vi "GUI Open Synchronization Objects.vi"(8 "error in (no error)":errorcluster) -> (0 "error out":errorcluster, 3 "FOFB GUI":T1)   [LabVIEW 2011, in "User Interface VIs.lvlib"]
uses:
  User Interface VIs.lvlib
  Types Definitions/Type FOFB GUI.ctl
  Types Definitions/Type FOFB Parameters.ctl
  Types Definitions/Type Network Configuration.ctl
  Types Definitions/Type FA Configuration.ctl
  Types Definitions/Type Response Matrix Measurement Configuration.ctl
  Types Definitions/Type Correction Algorithm Configuration.ctl
  Types Definitions/Type Acquisition Network Configuration.ctl
  Types Definitions/Type Actuation Network Configuration.ctl
  Types Definitions/Type Configuration Loop Mode.ctl
  Types Definitions/Type Configuration Data (GUI to Controller).ctl
  Types Definitions/Type Monitoring Data.ctl
  Types Definitions/Type Diagnostics Data.ctl
  Types Definitions/Type CPU Loads Array.ctl
  Types Definitions/Type CPU Loads.ctl
  Types Definitions/Type Diagnostics Sample.ctl
  Types Definitions/Type Monitoring Sample.ctl
  Type Definitions.lvlib
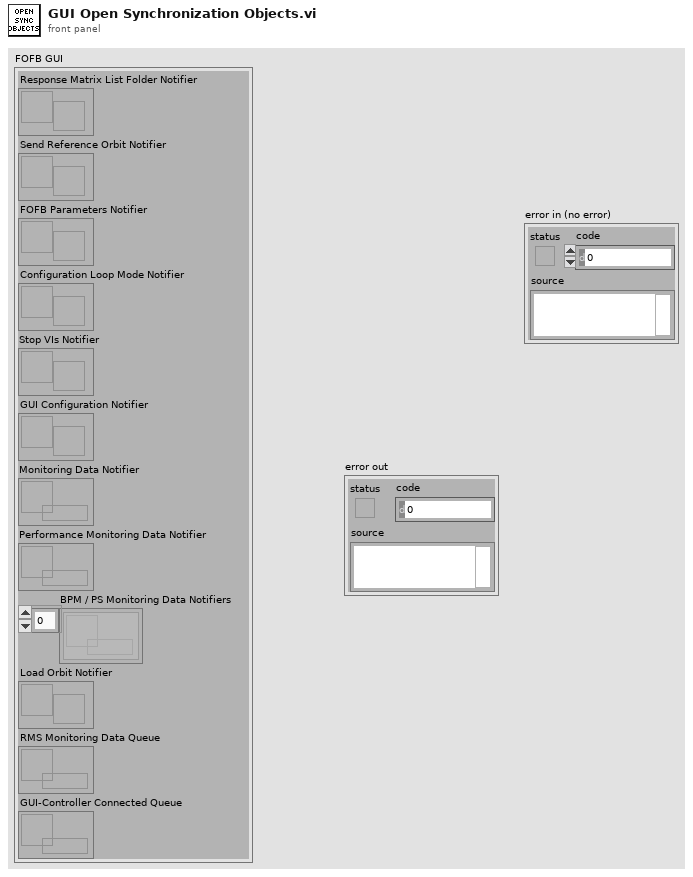
[diagram p1: front panel]
types:
  T1 = typedef "Type Definitions.lvlib/Type FOFB GUI.ctl" = cluster{"Response Matrix List Folder Notifier":refnum<notifier>, "Send Reference Orbit Notifier":refnum<notifier>, "FOFB Parameters Notifier":refnum<notifier>, "Configuration Loop Mode Notifier":refnum<notifier>, "Stop VIs Notifier":refnum<notifier>, "GUI Configuration Notifier":refnum<notifier>, "Monitoring Data Notifier":refnum<queue>, "Performance Monitoring Data Notifier":refnum<queue>, "BPM / PS Monitoring Data Notifiers":refnum<queue>[], "Load Orbit Notifier":refnum<notifier>, "RMS Monitoring Data Queue":refnum<queue>, "GUI-Controller Connected Queue":refnum<queue>}
  T2 = typedef "Type Definitions.lvlib/Type Configuration Loop Mode.ctl" = enum8{"Operation Mode", "Request FOFB Parameters", "Send New FOFB Parameters", "Send Reference Orbit", "Request Response Matrix List Folder"}
  T3 = typedef "Type Definitions.lvlib/Type FOFB Parameters.ctl" = cluster{"Network":T4, "Fast Acquisition":T5, "Response Matrix Measurement":T6, "Correction Algorithm":T7, "Acquisition Network":T8, "Actuation Network":T9}
  T4 = typedef "Type Definitions.lvlib/Type Network Configuration.ctl" = cluster{"FOFB Controller IP":string, "LNLS Control Network IP":string, "LNLS Control Network Power Supplies TCP Port":u16, "LNLS Control Network FOFB Configuration TCP Port":u16, "Data Server TCP Port":u16, "Monitoring Data TCP Port":u16, "Configuration GUI TCP Port":u16, "TCP Listening Timeout":i32}
  T5 = typedef "Type Definitions.lvlib/Type FA Configuration.ctl" = cluster{"Acquisition Period":u32, "Data Buffer Size":u32, "Monitoring Period":u32}
  T6 = typedef "Type Definitions.lvlib/Type Response Matrix Measurement Configuration.ctl" = cluster{"Step Amplitude":dbl, "Time Between Steps":u32, "Step Duration":u32, "Number of Averages":u32}
  T7 = typedef "Type Definitions.lvlib/Type Correction Algorithm Configuration.ctl" = cluster{"Correction Period":u32, "Reference Orbit Path":path, "Response Matrix Path":path, "Correction Matrix Path":path, "Horizontal Correction Factor":dbl, "Vertical Correction Factor":dbl, "Beam Current FOFB Threshold":dbl, "Decouple H-V":bool, "Use Additional BPM LPF":bool, "BPM LPF Cutoff":dbl}
  T8 = typedef "Type Definitions.lvlib/Type Acquisition Network Configuration.ctl" = cluster{"Chassis Name":string, "Variables":cluster{"Variable Name":string, "Matrix Order":u32, "Location":dbl, "Plane":enum8{"H", "V"}, "On Correction":bool}[]}[]
  T9 = typedef "Type Definitions.lvlib/Type Actuation Network Configuration.ctl" = cluster{"Chassis Name":string, "Variables":cluster{"Variable Name":string, "Matrix Order":u32, "RMM Step Factor":dbl, "Plane":enum8{"H", "V"}, "On Correction":bool, "Kc":dbl, "Ti":dbl, "Td":dbl}[]}[]
  T10 = typedef "Type Definitions.lvlib/Type Configuration Data (GUI to Controller).ctl" = cluster{"Update Controller Soft Configuration":bool[], "Request RT Execution Trace":string[], "Reference Orbit":dbl[], "Request Response Matrix Folder List":bool[], "Request FOFB Parameters":bool[], "FOFB Parameters":T3[]}
  T11 = typedef "Type Definitions.lvlib/Type Diagnostics Sample.ctl" = cluster{"Timestamp":timestamp, "Diagnostics Data":T12}
  T12 = typedef "Type Definitions.lvlib/Type Diagnostics Data.ctl" = cluster{"Time-Critical Loop Missed Iterations":u32, "Time-Critical Loop Execution Time (usec)":u32, "FA Buffer Usage":u32, "Available Memory (bytes)":u32, "CPU Loads Array":T13}
  T13 = typedef "Type Definitions.lvlib/Type CPU Loads Array.ctl" = T14[]
  T14 = typedef "Type Definitions.lvlib/Type CPU Loads.ctl" = cluster{"Total (%)":dbl, "Time Critical (%)":dbl, "Timed Structures (%)":dbl, "High (%)":dbl, "Above Normal (%)":dbl, "Normal (%)":dbl, "Background (%)":dbl, "Idle (%)":dbl, "ISR (%)":dbl}
  T15 = typedef "Type Definitions.lvlib/Type Monitoring Sample.ctl" = cluster{"Timestamp":timestamp, "Sample":dbl[]}
  T16 = typedef "Type Definitions.lvlib/Type Monitoring Data.ctl" = cluster{"Timestamp":timestamp, "BPM Readings":dbl[], "PS Readings":dbl[], "PS FOFB Setpoints":dbl[], "PS Status per Rack":u8[], "PS ON-OFF per Rack":u8[], "Operation Mode":enum16{"Idle Mode", "Error Mode", "Manual Mode", "FOFB Mode", "RMM Mode"}, "Diagnostics Data":T12, "Controller Status Table":i32[]}
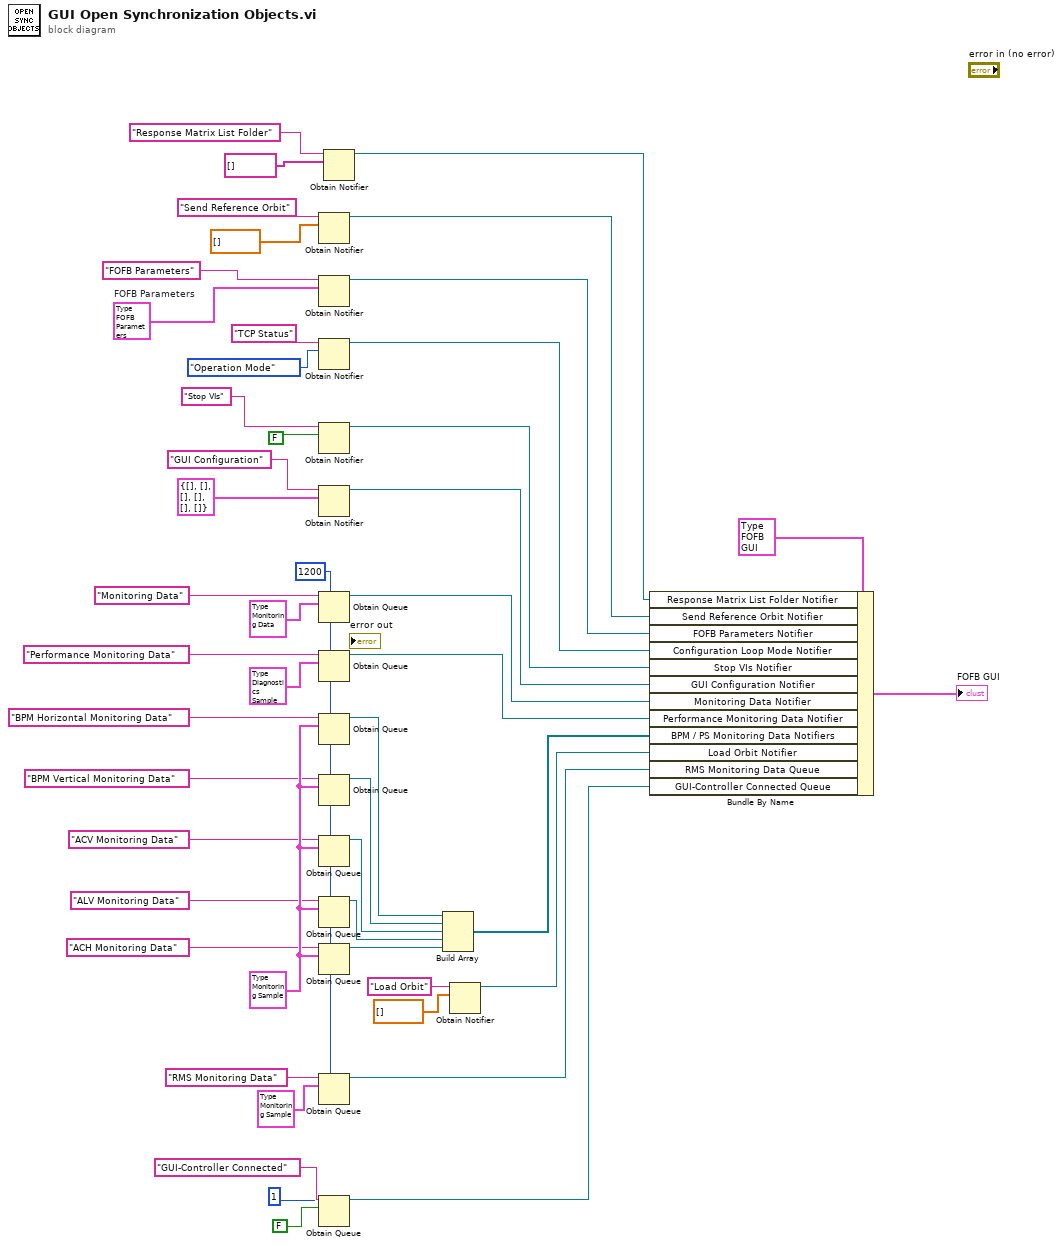
[diagram p0: block diagram]
diagram:
  w10 = T3 {"Network"={"FOFB Controller IP"="", "LNLS Control Network IP"="", "LNLS Control Network Power Supplies TCP Port"=0, "LNLS Control Network FOFB Configuration TCP Port"=0, "Data Server TCP Port"=0, "Monitoring Data TCP Port"=0, "Configuration GUI TCP Port"=0, "TCP Listening Timeout"=0}, "Fast Acquisition"={"Acquisition Period"=0, "Data Buffer Size"=0, "Monitoring Period"=0}, "Response Matrix Measurement"={"Step Amplitude"=0.0, "Time Between Steps"=0, "Step Duration"=0, "Number of Averages"=0}, "Correction Algorithm"={"Correction Period"=0, "Reference Orbit Path"=path "", "Response Matrix Path"=path "", "Correction Matrix Path"=path "", "Horizontal Correction Factor"=0.0, "Vertical Correction Factor"=0.0, "Beam Current FOFB Threshold"=0.0, "Decouple H-V"=FALSE, "Use Additional BPM LPF"=FALSE, "BPM LPF Cutoff"=0.0}, "Acquisition Network"=[], "Actuation Network"=[]}  # FOFB Parameters
  w37 = T15 {"Timestamp"=timestamp(0 s since 1904-01-01), "Sample"=[]} ("Monitoring Sample")
  w13 = 1200 ("max queue size (-1, unlimited)")
  n1 = Obtain Notifier(name (unnamed)="Send Reference Orbit", notification data type=dbl[] [] ("Orbit")) -> (notifier out=w5:refnum<notifier>)  [unwired: 2 in, 2 out]
  n2 = Obtain Notifier(name (unnamed)="FOFB Parameters", notification data type=w10) -> (notifier out=w9:refnum<notifier>)  [unwired: 2 in, 2 out]
  n3 = Obtain Notifier(name (unnamed)="TCP Status", notification data type=Type_Configuration_Loop_Mode."Operation Mode" ("notification")) -> (notifier out=w8:refnum<notifier>)  [unwired: 2 in, 2 out]
  n4 = Obtain Notifier(name (unnamed)="Stop VIs", notification data type=FALSE) -> (notifier out=w41:refnum<notifier>)  [unwired: 2 in, 2 out]
  n5 = Obtain Notifier(name (unnamed)="GUI Configuration", notification data type=T10 {"Update Controller Soft Configuration"=[], "Request RT Execution Trace"=[], "Reference Orbit"=[], "Request Response Matrix Folder List"=[], "Request FOFB Parameters"=[], "FOFB Parameters"=[]} ("Configuration Data (GUI to Controller)")) -> (notifier out=w42:refnum<notifier>)  [unwired: 2 in, 2 out]
  n6 = Obtain Queue(max queue size (-1, unlimited)=w13, name (unnamed)="Monitoring Data", element data type=T16 {"Timestamp"=timestamp(0 s since 1904-01-01), "BPM Readings"=[], "PS Readings"=[], "PS FOFB Setpoints"=[], "PS Status per Rack"=[], "PS ON-OFF per Rack"=[], "Operation Mode"=enum."Idle Mode", "Diagnostics Data"={"Time-Critical Loop Missed Iterations"=0, "Time-Critical Loop Execution Time (usec)"=0, "FA Buffer Usage"=0, "Available Memory (bytes)"=0, "CPU Loads Array"=[]}, "Controller Status Table"=[]} ("Slow Data")) -> (queue out=w43:refnum<queue>)  [unwired: 2 in, 2 out]
  n7 = Obtain Queue(max queue size (-1, unlimited)=w13, name (unnamed)="Performance Monitoring Data", element data type=T11 {"Timestamp"=timestamp(0 s since 1904-01-01), "Diagnostics Data"={"Time-Critical Loop Missed Iterations"=0, "Time-Critical Loop Execution Time (usec)"=0, "FA Buffer Usage"=0, "Available Memory (bytes)"=0, "CPU Loads Array"=[]}} ("Diagnostics  Sample")) -> (queue out=w44:refnum<queue>)  [unwired: 2 in, 2 out]
  n8 = Obtain Queue(max queue size (-1, unlimited)=w13, name (unnamed)="BPM Horizontal Monitoring Data", element data type=w37) -> (queue out=w30:refnum<queue>)  [unwired: 2 in, 2 out]
  n9 = Obtain Queue(max queue size (-1, unlimited)=w13, name (unnamed)="BPM Vertical Monitoring Data", element data type=w37) -> (queue out=w31:refnum<queue>)  [unwired: 2 in, 2 out]
  n10 = Obtain Queue(max queue size (-1, unlimited)=w13, name (unnamed)="ACV Monitoring Data", element data type=w37) -> (queue out=w32:refnum<queue>)  [unwired: 2 in, 2 out]
  n11 = Obtain Queue(max queue size (-1, unlimited)=w13, name (unnamed)="ALV Monitoring Data", element data type=w37) -> (queue out=w33:refnum<queue>)  [unwired: 2 in, 2 out]
  n12 = Obtain Queue(max queue size (-1, unlimited)=w13, name (unnamed)="ACH Monitoring Data", element data type=w37) -> (queue out=w36:refnum<queue>)  [unwired: 2 in, 2 out]
  n13 = Obtain Queue(max queue size (-1, unlimited)=w13, name (unnamed)="RMS Monitoring Data", element data type=T15 {"Timestamp"=timestamp(0 s since 1904-01-01), "Sample"=[]} ("Monitoring Sample")) -> (queue out=w49:refnum<queue>)  [unwired: 2 in, 2 out]
  n14 = Obtain Queue(max queue size (-1, unlimited)=1, name (unnamed)="GUI-Controller Connected", element data type=FALSE) -> (queue out=w16:refnum<queue>)  [unwired: 2 in, 2 out]
  n15 = Obtain Notifier(name (unnamed)="Response Matrix List Folder", notification data type=string[] [] ("Request Response Matrix List Folder")) -> (notifier out=w1:refnum<notifier>)  [unwired: 2 in, 2 out]
  n16 = Build Array(w30, w31, w32, w33, w36) -> (w45:refnum<queue>[])
  n17 = Obtain Notifier(name (unnamed)="Load Orbit", notification data type=dbl[] [] ("initialized array")) -> (notifier out=w48:refnum<notifier>)  [unwired: 2 in, 2 out]
  n18 = Bundle By Name(cluster=T1 {"Response Matrix List Folder Notifier"=refnum, "Send Reference Orbit Notifier"=refnum, "FOFB Parameters Notifier"=refnum, "Configuration Loop Mode Notifier"=refnum, "Stop VIs Notifier"=refnum, "GUI Configuration Notifier"=refnum, "Monitoring Data Notifier"=refnum, "Performance Monitoring Data Notifier"=refnum, "BPM / PS Monitoring Data Notifiers"=[], "Load Orbit Notifier"=refnum, "RMS Monitoring Data Queue"=refnum, "GUI-Controller Connected Queue"=refnum} ("FOFB GUI"), "Response Matrix List Folder Notifier"=w1, "Send Reference Orbit Notifier"=w5, "FOFB Parameters Notifier"=w9, "Configuration Loop Mode Notifier"=w8, "Stop VIs Notifier"=w41, "GUI Configuration Notifier"=w42, "Monitoring Data Notifier"=w43, "Performance Monitoring Data Notifier"=w44, "BPM / PS Monitoring Data Notifiers"=w45, "Load Orbit Notifier"=w48, "RMS Monitoring Data Queue"=w49, "GUI-Controller Connected Queue"=w16) -> (→"FOFB GUI":T1)
